vi "ClassRelationshipEdge_Create.vi"(0 "reference":refnum<class "ClassRelationshipEdge.lvclass">, 5 "error in (no error)":errorcluster) -> (14 "reference out":refnum<class "ClassRelationshipEdge.lvclass">, 16 "# of objects":i32, 19 "error out":errorcluster)   [LabVIEW 2014, in "ClassRelationshipEdge.lvclass"]
doc: "Creates and initializes a new ClassRelationshipEdge object.\n\nThis object should be destroyed using a ClassRelationshipEdge destructor VI or a virtual base class destructor VI.\n\n[GOOP 2.1]"
uses:
  <resource>/Framework/Providers/Open_GDS/UML/ClassRelationshipEdge_class/ClassRelationshipEdge.lvclass
  <resource>/Framework/Providers/Open_GDS/UML/BentStyle_class/BentStyleType.ctl
  <resource>/Framework/Providers/Open_GDS/UML/SegmentedLineEdge_class/SegmentedLineEdge.lvclass
  <resource>/Framework/Providers/Open_GDS/UML/BentStyle_class/BentStyle.lvclass
panel:
  # "The input reference should only\nbe wired when this method is called\nby a sub class constructor."
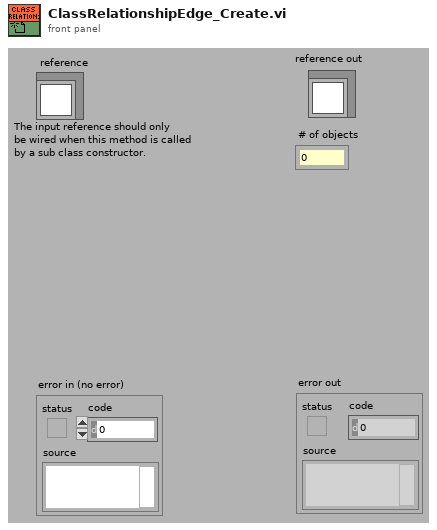
[diagram p1: front panel]
types:
  T1 = typedef "BentStyle.lvclass/BentStyleType.ctl" = enum16{"STRAIGHT", "HV", "VH", "HVH", "VHV", "ARC"}
  T2 = typedef "ClassRelationshipEdge.lvclass/ObjectAttributes.ctl" = cluster{"bentStyleRef":refnum<class "BentStyle.lvclass">, "startConnectionOffset":cluster{"x":i32, "y":i32}, "endConnectionOffset":cluster{"x":i32, "y":i32}, "MidLineOffset":cluster{"x":i32, "y":i32}, "DepClass":T3}
  T3 = typedef "ReversedEngineering_ViDependencyDetailsType.ctl" = cluster{"ThisVIs/Ctls":path[], "Dependent_VIs/Ctls":path[]}
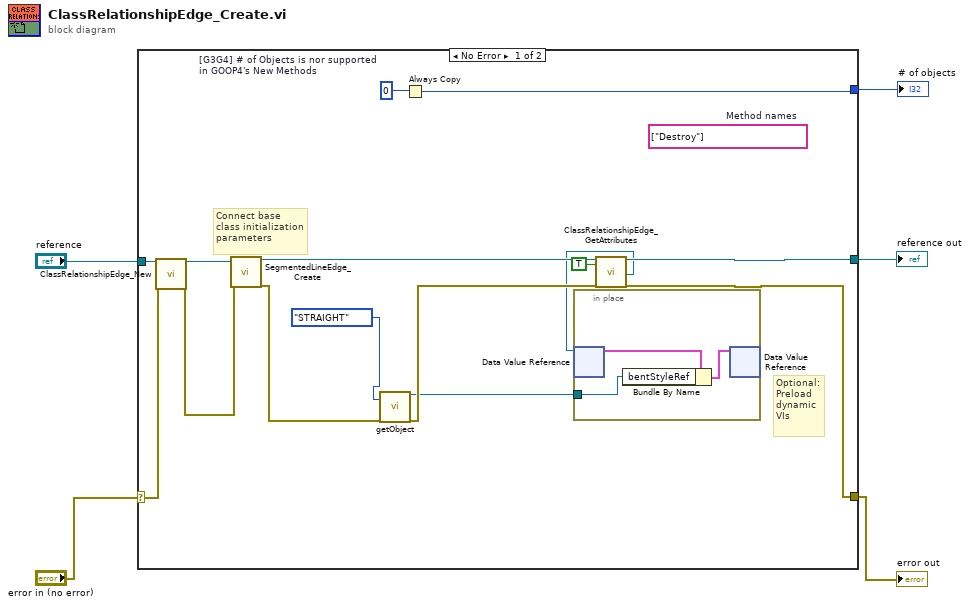
[diagram p0: block diagram]
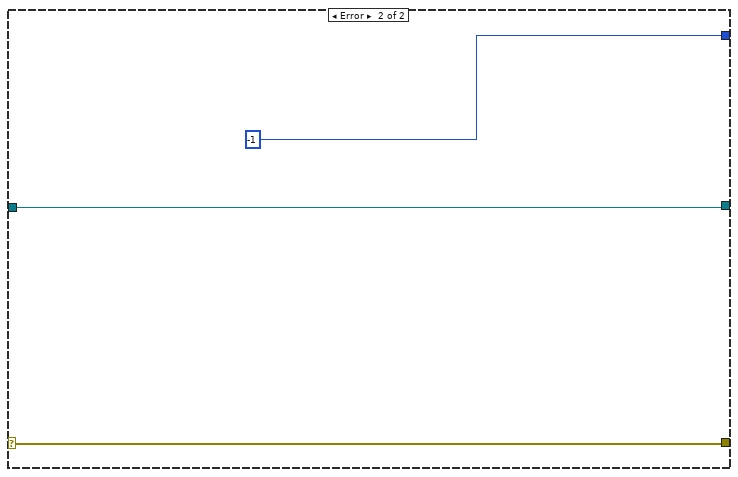
[diagram p2: hidden frame]
diagram:
  n1 = case shown="No Error" "error in (no error)" {
    selector: "error in (no error)" -> [w20 w25]
    tunnel: [w15 w24] -> w5
    tunnel: [w14 w25] -> w4
    tunnel: [w10 -1 ("Nr of open handles")] -> w3
    tunnel: "reference" -> [w19 w24]
    frame No Error {
      w6 = 0  # [G3G4] # of Objects is nor supported in GOOP4's New Methods
      (unwired) string[] ["Destroy"]  # Method names
      # "Optional:\nPreload\ndynamic\nVIs"
      # "Connect base\nclass initialization\nparameters"
      n2 = call <resource>:"ClassRelationshipEdge_New.vi"("reference in"=w19, "error in (no error)"=w20) -> ("reference out"=w17:refnum<class "ClassRelationshipEdge.lvclass">, "error out"=w18:errorcluster)  [unwired: 2 in, 14 out]
      n3 = call <resource>:"SegmentedLineEdge_Create.vi"("reference"=w17, "error in (no error)"=w18) -> ("reference out"=w16:refnum<class "ClassRelationshipEdge.lvclass">, "error out"=w12:errorcluster)  [unwired: 1 in, 15 out]
      n4 = call <resource>:"getObject.vi"("bentStyle"=BentStyleType."STRAIGHT", "error in (no error)"=w12) -> ("reference out"=w7:refnum<class "BentStyle.lvclass">, "error out"=w11:errorcluster)  [unwired: 16 out]
      n5 = Always Copy(1:w6) -> (0:w10:i32)
      n6 = call <resource>:"ClassRelationshipEdge_GetAttributes.vi"("reference in"=w16, "OnlyGetDvrReference(False)"=TRUE, "error in (no error)"=w11) -> ("reference out"=w15:refnum<class "ClassRelationshipEdge.lvclass">, "DataRef"=w8:refnum<data-value>, "error out"=w14:errorcluster)  [unwired: 13 in, 1 out]
      n7 = in-place {
        in-place-border: w7 -> [w22]
        n8 = in-place-dvr #1(w8) -> (w23:T2)  [unwired: 1 out]
        n9 = Bundle By Name(cluster=w23, "bentStyleRef"=w22) -> (w21:T2)
        n10 = in-place-dvr #1(w21) -> ()  [unwired: 2 out]
      }
    }
    frame Error {
    }
  }
  "error out" <- w4
  "reference out" <- w5
  "# of objects" <- w3
